vi "MOVE2.vi"(1 "Relative":bool, 2 "Position to go":T1={"X"=FALSE, "Target X (um)"=1000.0, "Current X (um)"=1000.0, "Scaling X"=0, "Y"=FALSE, "Target Y (um)"=0.0, "Current Y (um)"=0.0, "Scaling Y"=0, "Z"=FALSE, "Target Z (um)"=0.0, "Current Z (um)"=0.0, "Scaling Z"=0} {"Current X (um)" step=1.0; "Scaling Z" items=["X", "Z", "None"]; "Scaling Y" items=["X", "Z", "None"]; "Scaling X" items=["X", "Z", "None"]; "Target X (um)" step=1.0}) -> (0 "command":string)   [LabVIEW 2018]
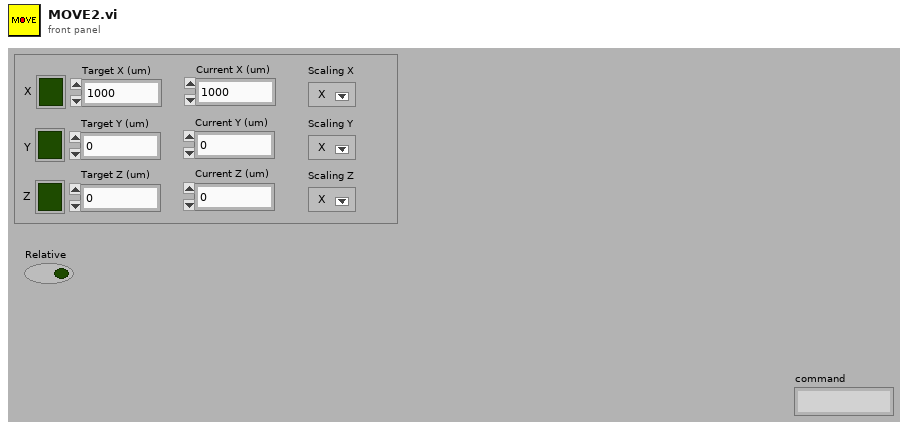
[diagram p1: front panel]
types:
  T1 = cluster{"X":bool, "Target X (um)":dbl, "Current X (um)":dbl, "Scaling X":u16, "Y":bool, "Target Y (um)":dbl, "Current Y (um)":dbl, "Scaling Y":u16, "Z":bool, "Target Z (um)":dbl, "Current Z (um)":dbl, "Scaling Z":u16}
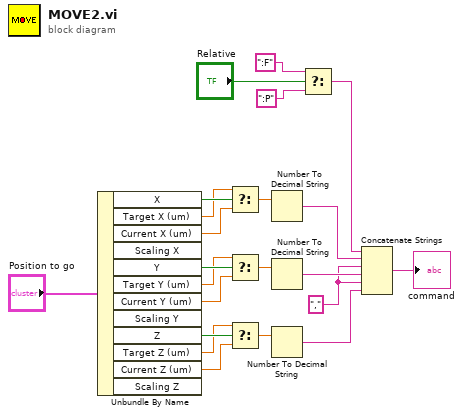
[diagram p0: block diagram]
diagram:
  w20 = ","
  n1 = Unbundle By Name("Position to go") -> ("X"=w13:bool, "Target X (um)"=w9:dbl, "Current X (um)"=w8:dbl, "Y"=w12:bool, "Target Y (um)"=w7:dbl, "Current Y (um)"=w6:dbl, "Z"=w11:bool, "Target Z (um)"=w5:dbl, "Current Z (um)"=w4:dbl)  [unwired: 3 out]
  n2 = Select(t=w9, s=w13, f=w8) -> (s? t:f=w3:dbl)
  n3 = Select(t=w7, s=w12, f=w6) -> (s? t:f=w2:dbl)
  n4 = Select(t=w5, s=w11, f=w4) -> (s? t:f=w1:dbl)
  n5 = Number To Decimal String(number=w3) -> (decimal integer string=w22:string)  [unwired: 1 in]
  n6 = Number To Decimal String(number=w2) -> (decimal integer string=w21:string)  [unwired: 1 in]
  n7 = Number To Decimal String(number=w1) -> (decimal integer string=w19:string)  [unwired: 1 in]
  n8 = Select(t=":F", s="Relative", f=":P") -> (s? t:f=w15:string)
  n9 = Concatenate Strings(w15, w22, w20, w21, w20, w19) -> (→"command":string)
